vi "LEDC Control Loop 1931 Main 2.vi"(0 "LEDAD Port":refnum<visa-resource-name>="COM9", 1 "Enable":u8, 2 "Inten Desired":refnum<vi>, 3 "Illum Meas":refnum<vi>, 5 "Light Meter Port":refnum<visa-resource-name>="COM3", 7 "Illum Desired":dbl, 9 "Error Margin":dbl=2.0, 11 "error in (no error)":errorcluster, 12 "Illum Cal Factor":dbl=0.444212 format="%#.6f", 13 "Zero Adj":dbl) -> (4 "LEDAD Port out":refnum<visa-resource-name>, 6 "Light Meter Port out":refnum<visa-resource-name>, 8 "Illum Meas":dbl format="%#_4g", 10 "Inten Desired":dbl, 14 "Done":bool, 15 "error out":errorcluster)   [LabVIEW 2010]
panel:
  out "Flag2":bool
  out "Flag1":bool
  out "Slope":dbl format="%#_4g"
  in  "Illum 10":dbl format="%#_4g"
  in  "Stop":bool
  out "In Progress":bool
  in  "Illum 90":dbl format="%#_4g"
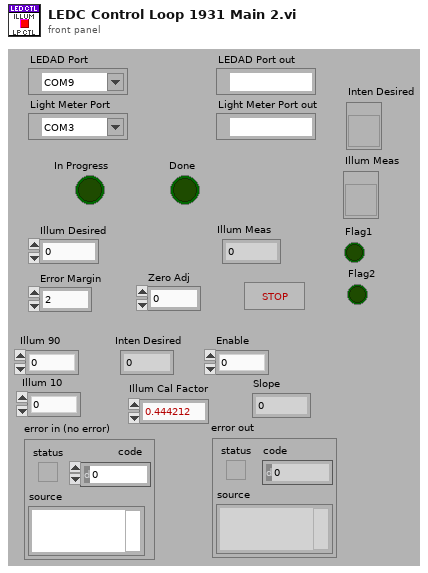
[diagram p1: front panel]
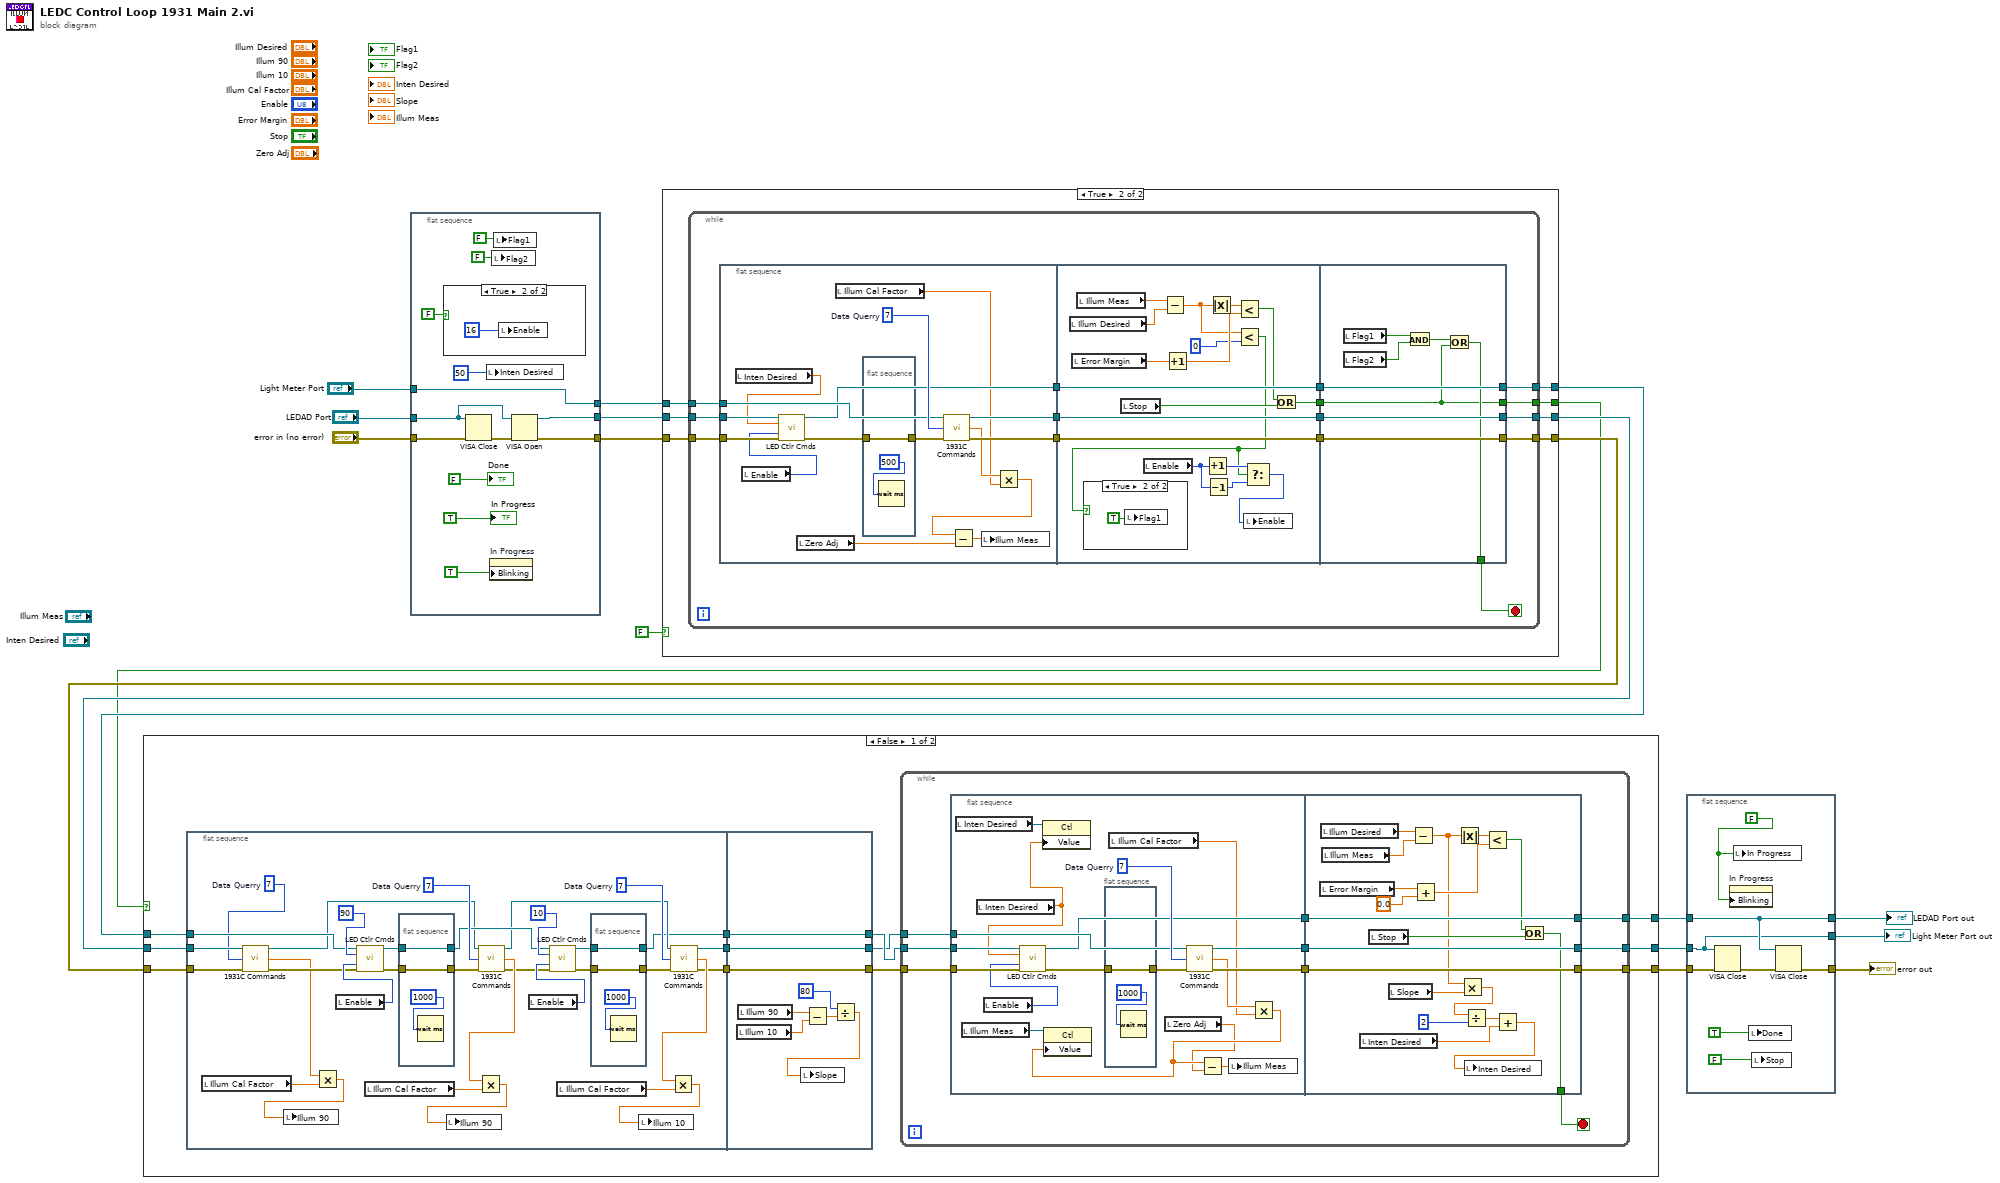
[diagram p0: block diagram]
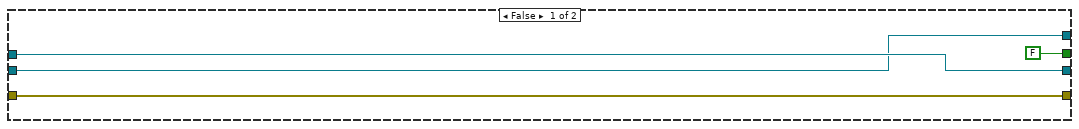
[diagram p2: hidden frame]
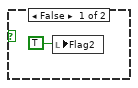
[diagram p3: hidden frame]
diagram:
  n1 = flat-sequence {
    tunnel: "LEDAD Port" -> [w23]
    tunnel: [w25] -> w14
    tunnel: "error in (no error)" -> [w26]
    tunnel: [w24] -> w16
    tunnel: "Light Meter Port" -> [w22]
    tunnel: [w22] -> w15
    frame #0 {
      n2 = case shown="True" FALSE {
        frame False {
        }
        frame True {
          n3 = local write "Enable"(16) -> ()
        }
      }
      n4 = VISA Close(VISA resource name=w23, error in (no error)=w26) -> (error out=w27:errorcluster)
      n5 = local write "Inten Desired"(50) -> ()
      n6 = property on="In Progress" class="Bool (strict)"("Blinking"=TRUE) -> ()  [unwired: 2 in, 2 out]
      n7 = local write "Flag2"(FALSE) -> ()
      n8 = local write "Flag1"(FALSE) -> ()
      n9 = VISA Open(error in (no error)=w27, VISA resource name=w23) -> (VISA resource name=w24:refnum<visa-resource-name>, error out=w25:errorcluster)  [unwired: 3 in]
      "Done" <- FALSE
      "In Progress" <- TRUE
    }
  }
  n10 = case shown="True" FALSE {
    tunnel: w16 -> [w34 w42]
    tunnel: w15 -> [w35 w41]
    tunnel: w14 -> [w33 w40]
    tunnel: [w34 w39] -> w10
    tunnel: [w35 w38] -> w9
    tunnel: [w33 w37] -> w8
    tunnel: [FALSE w36] -> w7
    frame False {
    }
    frame True {
      n11 = while {
        tunnel: w41 -> [w57]
        tunnel: w42 -> [w56]
        tunnel: w40 -> [w55]
        tunnel: [w48] -> w38
        tunnel: [w46] -> w37
        tunnel: [w47] -> w39
        tunnel: [w43] -> w36
        stop <- w44 stop-if-true
        n12 = flat-sequence {
          tunnel: w55 -> [w71]
          tunnel: w56 -> [w72]
          tunnel: w57 -> [w70]
          tunnel: [w69] -> w51
          tunnel: [w67] -> w50
          tunnel: [w68] -> w49
          tunnel: [w92] -> w54
          tunnel: [w91] -> w53
          tunnel: [w90] -> w52
          tunnel: w51 -> [w92]
          tunnel: w50 -> [w91]
          tunnel: w49 -> [w90]
          tunnel: [w77] -> w45
          tunnel: w54 -> [w103]
          tunnel: w53 -> [w102]
          tunnel: w52 -> [w101]
          tunnel: [w103] -> w48
          tunnel: [w102] -> w47
          tunnel: [w101] -> w46
          tunnel: w45 -> [w96]
          tunnel: [w97] -> w44
          tunnel: [w96] -> w43
          frame #0 {
            w73 = 7  # Data Querry
            n13 = local read "Inten Desired"() -> (w64:dbl)
            n14 = local read "Enable"() -> (w63:u8)
            n15 = call "LED Ctlr Cmds.vi"("VISA session"=w72, "Intensity"=w64, "Enable"=w63, "error in (no error)"=w71) -> ("VISA session out"=w67:refnum<visa-resource-name>, "error out"=w66:errorcluster)  [unwired: 7 in, 3 out]
            n16 = local read "Zero Adj"() -> (w58:dbl)
            n17 = local read "Illum Cal Factor"() -> (w61:dbl)
            n18 = flat-sequence {
              tunnel: w66 -> [w75]
              tunnel: [w75] -> w65
              frame #0 {
                n19 = Wait (ms)(milliseconds to wait=500) -> ()  [unwired: 1 out]
              }
            }
            n20 = call "1931C Commands.vi"("Instrument Resource Name"=w70, "Command"=w73, "error in (no error)"=w65) -> ("VISA resource name out"=w69:refnum<visa-resource-name>, "LM Response"=w62:dbl, "error out"=w68:errorcluster)  [unwired: 8 in, 2 out]
            n21 = Multiply(x=w62, y=w61) -> (x*y=w59:dbl)
            n22 = Subtract(x=w59, y=w58) -> (x-y=w60:dbl)
            n23 = local write "Illum Meas"(w60) -> ()
          }
          frame #1 {
            n24 = local read "Illum Desired"() -> (w87:dbl)
            n25 = local read "Error Margin"() -> (w85:dbl)
            n26 = local read "Illum Meas"() -> (w88:dbl)
            n27 = local read "Stop"() -> (w84:bool)
            n28 = local read "Enable"() -> (w79:u8)
            n29 = Subtract(x=w88, y=w87) -> (x-y=w83:dbl)
            n30 = Increment(x=w85) -> (x+1=w86:dbl)
            n31 = Increment(x=w79) -> (x+1=w80:u8)
            n32 = Decrement(x=w79) -> (x-1=w81:u8)
            n33 = Absolute Value(x=w83) -> (abs(x)=w93:dbl)
            n34 = Less?(x=w93, y=w86) -> (x < y?=w89:bool)
            n35 = Less?(x=w83, y=0) -> (x < y?=w78:bool)
            n36 = case shown="True" w78 {
              frame False {
                n37 = local write "Flag2"(TRUE) -> ()
              }
              frame True {
                n38 = local write "Flag1"(TRUE) -> ()
              }
            }
            n39 = Select(t=w80, s=w78, f=w81) -> (s? t:f=w76:u8)
            n40 = local write "Enable"(w76) -> ()
            n41 = Or(x=w89, y=w84) -> (x .or. y?=w77:bool)
          }
          frame #2 {
            n42 = local read "Flag1"() -> (w100:bool)
            n43 = local read "Flag2"() -> (w99:bool)
            n44 = And(x=w100, y=w99) -> (x .and. y?=w98:bool)
            n45 = Or(x=w98, y=w96) -> (x .or. y?=w97:bool)
          }
        }
      }
    }
  }
  n46 = case shown="False" w7 {
    tunnel: w10 -> [w107 w212]
    tunnel: w9 -> [w113 w213]
    tunnel: w8 -> [w112 w214]
    tunnel: [w108 w214] -> w6
    tunnel: [w110 w213] -> w5
    tunnel: [w109 w212] -> w4
    frame False {
      n47 = flat-sequence {
        tunnel: w113 -> [w123]
        tunnel: w112 -> [w122]
        tunnel: [w129] -> w115
        tunnel: [w128] -> w114
        tunnel: w107 -> [w127]
        tunnel: [w124] -> w106
        tunnel: [w162] -> w104
        tunnel: w115 -> [w162]
        tunnel: [w161] -> w111
        tunnel: w114 -> [w161]
        tunnel: [w157] -> w105
        tunnel: w106 -> [w157]
        frame #0 {
          w119 = 7  # Data Querry
          w136 = 7  # Data Querry
          w143 = 7  # Data Querry
          n48 = local read "Illum Cal Factor"() -> (w118:dbl)
          n49 = call "1931C Commands.vi"("Instrument Resource Name"=w123, "Command"=w119, "error in (no error)"=w122) -> ("VISA resource name out"=w121:refnum<visa-resource-name>, "LM Response"=w116:dbl, "error out"=w120:errorcluster)  [unwired: 8 in, 2 out]
          n50 = Multiply(x=w116, y=w118) -> (x*y=w117:dbl)
          n51 = local write "Illum 90"(w117) -> ()
          n52 = local read "Enable"() -> (w148:u8)
          n53 = call "LED Ctlr Cmds.vi"("VISA session"=w127, "Intensity"=90, "Enable"=w148, "error in (no error)"=w120) -> ("VISA session out"=w145:refnum<visa-resource-name>, "error out"=w146:errorcluster)  [unwired: 7 in, 3 out]
          n54 = local read "Illum Cal Factor"() -> (w140:dbl)
          n55 = flat-sequence {
            tunnel: w146 -> [w154]
            tunnel: [w154] -> w144
            tunnel: [w152] -> w126
            tunnel: w145 -> [w152]
            frame #0 {
              n56 = Wait (ms)(milliseconds to wait=1000) -> ()  [unwired: 1 out]
            }
          }
          n57 = call "1931C Commands.vi"("Instrument Resource Name"=w121, "Command"=w143, "error in (no error)"=w144) -> ("VISA resource name out"=w125:refnum<visa-resource-name>, "LM Response"=w141:dbl, "error out"=w130:errorcluster)  [unwired: 8 in, 2 out]
          n58 = Multiply(x=w141, y=w140) -> (x*y=w142:dbl)
          n59 = local write "Illum 90"(w142) -> ()
          n60 = local read "Enable"() -> (w131:u8)
          n61 = call "LED Ctlr Cmds.vi"("VISA session"=w126, "Intensity"=10, "Enable"=w131, "error in (no error)"=w130) -> ("VISA session out"=w134:refnum<visa-resource-name>, "error out"=w133:errorcluster)  [unwired: 7 in, 3 out]
          n62 = local read "Illum Cal Factor"() -> (w139:dbl)
          n63 = flat-sequence {
            tunnel: w133 -> [w151]
            tunnel: [w151] -> w135
            tunnel: [w149] -> w124
            tunnel: w134 -> [w149]
            frame #0 {
              n64 = Wait (ms)(milliseconds to wait=1000) -> ()  [unwired: 1 out]
            }
          }
          n65 = call "1931C Commands.vi"("Instrument Resource Name"=w125, "Command"=w136, "error in (no error)"=w135) -> ("VISA resource name out"=w129:refnum<visa-resource-name>, "LM Response"=w138:dbl, "error out"=w128:errorcluster)  [unwired: 8 in, 2 out]
          n66 = Multiply(x=w138, y=w139) -> (x*y=w137:dbl)
          n67 = local write "Illum 10"(w137) -> ()
        }
        frame #1 {
          n68 = local read "Illum 10"() -> (w159:dbl)
          n69 = local read "Illum 90"() -> (w160:dbl)
          n70 = Subtract(x=w160, y=w159) -> (x-y=w156:dbl)
          n71 = Divide(x=80, y=w156) -> (x/y=w158:dbl)
          n72 = local write "Slope"(w158) -> ()
        }
      }
      n73 = while {
        tunnel: w104 -> [w172]
        tunnel: w105 -> [w171]
        tunnel: w111 -> [w170]
        tunnel: [w166] -> w110
        tunnel: [w164] -> w108
        tunnel: [w165] -> w109
        stop <- w163 stop-if-true
        n74 = flat-sequence {
          tunnel: w170 -> [w188]
          tunnel: w171 -> [w189]
          tunnel: w172 -> [w187]
          tunnel: [w186] -> w169
          tunnel: [w184] -> w168
          tunnel: [w185] -> w167
          tunnel: w169 -> [w210]
          tunnel: w168 -> [w209]
          tunnel: w167 -> [w208]
          tunnel: [w195] -> w163
          tunnel: [w210] -> w166
          tunnel: [w209] -> w165
          tunnel: [w208] -> w164
          frame #0 {
            w190 = 7  # Data Querry
            n75 = local read "Inten Desired"() -> (w178:refnum<vi>)
            n76 = local read "Illum Meas"() -> (w176:refnum<vi>)
            n77 = local read "Inten Desired"() -> (w177:dbl)
            n78 = local read "Enable"() -> (w181:u8)
            n79 = call "LED Ctlr Cmds.vi"("VISA session"=w189, "Intensity"=w177, "Enable"=w181, "error in (no error)"=w188) -> ("VISA session out"=w184:refnum<visa-resource-name>, "error out"=w183:errorcluster)  [unwired: 7 in, 3 out]
            n80 = property class="Ctl"(reference=w178, "Value"=w177) -> ()  [unwired: 1 in, 2 out]
            n81 = flat-sequence {
              tunnel: w183 -> [w192]
              tunnel: [w192] -> w182
              frame #0 {
                n82 = Wait (ms)(milliseconds to wait=1000) -> ()  [unwired: 1 out]
              }
            }
            n83 = local read "Illum Cal Factor"() -> (w179:dbl)
            n84 = local read "Zero Adj"() -> (w173:dbl)
            n85 = call "1931C Commands.vi"("Instrument Resource Name"=w187, "Command"=w190, "error in (no error)"=w182) -> ("VISA resource name out"=w186:refnum<visa-resource-name>, "LM Response"=w180:dbl, "error out"=w185:errorcluster)  [unwired: 8 in, 2 out]
            n86 = Multiply(x=w180, y=w179) -> (x*y=w174:dbl)
            n87 = property class="Ctl"(reference=w176, "Value"=w174) -> ()  [unwired: 1 in, 2 out]
            n88 = Subtract(x=w174, y=w173) -> (x-y=w175:dbl)
            n89 = local write "Illum Meas"(w175) -> ()
          }
          frame #1 {
            n90 = local read "Error Margin"() -> (w194:dbl)
            n91 = local read "Illum Desired"() -> (w206:dbl)
            n92 = local read "Illum Meas"() -> (w205:dbl)
            n93 = local read "Inten Desired"() -> (w197:dbl)
            n94 = local read "Stop"() -> (w203:bool)
            n95 = local read "Slope"() -> (w201:dbl)
            n96 = Subtract(x=w206, y=w205) -> (x-y=w199:dbl)
            n97 = Add(x=w194, y=0.0) -> (x+y=w204:dbl)
            n98 = Absolute Value(x=w199) -> (abs(x)=w211:dbl)
            n99 = Multiply(x=w199, y=w201) -> (x*y=w198:dbl)
            n100 = Divide(x=w198, y=2) -> (x/y=w200:dbl)
            n101 = Less?(x=w211, y=w204) -> (x < y?=w207:bool)
            n102 = Add(x=w200, y=w197) -> (x+y=w196:dbl)
            n103 = local write "Inten Desired"(w196) -> ()
            n104 = Or(x=w207, y=w203) -> (x .or. y?=w195:bool)
          }
        }
      }
    }
    frame True {
    }
  }
  n105 = flat-sequence {
    tunnel: w5 -> [w218]
    tunnel: w6 -> [w220]
    tunnel: [w219] -> w2
    tunnel: w4 -> [w219]
    tunnel: [w218] -> w3
    tunnel: [w216] -> w17
    frame #0 {
      w222 = FALSE
      n106 = VISA Close(VISA resource name=w218, error in (no error)=w220) -> (error out=w217:errorcluster)
      n107 = property on="In Progress" class="Bool (strict)"("Blinking"=w222) -> ()  [unwired: 2 in, 2 out]
      n108 = local write "In Progress"(w222) -> ()
      n109 = local write "Done"(TRUE) -> ()
      n110 = local write "Stop"(FALSE) -> ()
      n111 = VISA Close(VISA resource name=w219, error in (no error)=w217) -> (error out=w216:errorcluster)
    }
  }
  "error out" <- w17
  "Light Meter Port out" <- w3
  "LEDAD Port out" <- w2
